vi "Auto Tank Drive.vi"(10 "Right":dbl, 11 "Left":dbl) -> ()   [LabVIEW 2015]
uses:
  Robot Global Data.vi
  Common Code/Drivetrain Modes.ctl
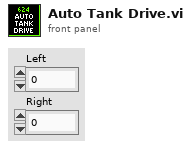
[diagram p1: front panel]
types:
  T1 = typedef "Drivetrain Modes.ctl" = enum16{"Climb", "Manual", "Goal Vision Targeting", "PID Distance Drive", "Hybrid", "Gyro Steer"}
  T2 = typedef "Drivetrain Commands.ctl" = cluster{"Y Power":dbl, "Turn Power":dbl, "Modes":T1, "Heading Target":dbl, "X Max Speed":dbl, "Y Max Speed":dbl, "X Min Speed":dbl, "Y Min Speed":dbl, "Y Target":dbl, "Max Accel":dbl, "Max Velocity":dbl, "Pivot Speed":dbl}
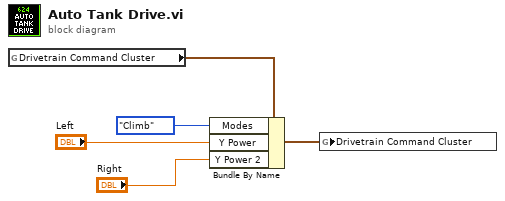
[diagram p0: block diagram]
diagram:
  n1 = global read "Robot Global Data.vi" "Drivetrain Command Cluster"() -> (w5:T2)
  n2 = Bundle By Name(cluster=w5, "Modes"=Drivetrain_Modes."Climb", "Y Power"="Left", "Y Power 2"="Right") -> (w3:T2)
  n3 = global write "Robot Global Data.vi" "Drivetrain Command Cluster"(w3) -> ()
